vi "Log State.vi"(8 "error in":errorcluster, 10 "Model Status":T3, 11 "Data":T1) -> (0 "error out":errorcluster, 3 "Data out":T1)   [LabVIEW 2015, in "Logger.lvlib"]
uses:
  Logger.lvlib
  Model/TypeDefs/Get Model Status Control.ctl
  TypeDefs/Logger Data.ctl
  TypeDefs/Logger State.ctl
  Model/Model.lvlib
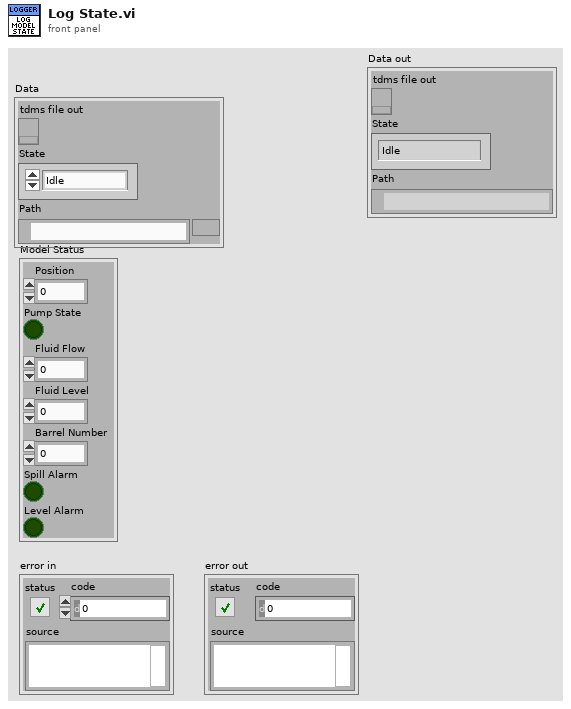
[diagram p1: front panel]
types:
  T1 = typedef "Logger.lvlib/Logger Data.ctl" = cluster{"tdms file out":refnum<k34>, "State":T2, "Path":path}
  T2 = typedef "Logger.lvlib/Logger State.ctl" = enum16{"Idle", "Working"}
  T3 = typedef "Model.lvlib/Get Model Status Control.ctl" = cluster{"Position":dbl, "Pump State":bool, "Fluid Flow":dbl, "Fluid Level":dbl, "Barrel Number":i32, "Spill Alarm":bool, "Level Alarm":bool}
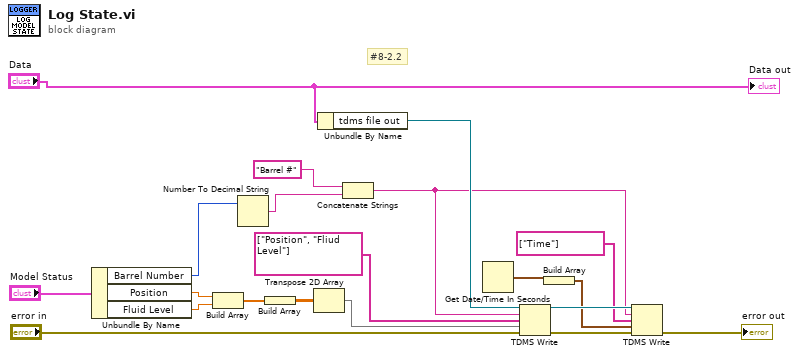
[diagram p0: block diagram]
diagram:
  # "#8-2.2"
  n1 = Unbundle By Name("Model Status") -> ("Barrel Number"=w14:i32, "Position"=w8:dbl, "Fluid Level"=w7:dbl)
  n2 = Build Array(w8, w7) -> (w6:dbl[])
  n3 = Number To Decimal String(number=w14) -> (decimal integer string=w13:string)  [unwired: 1 in]
  n4 = Build Array(w6) -> (w5:dbl[][])
  n5 = Transpose 2D Array(2D array=w5) -> (transposed array=w4:dbl[][])
  n6 = Unbundle By Name("Data") -> ("tdms file out"=w17:refnum<k34>)
  n7 = Concatenate Strings("Barrel #" ("string"), w13) -> (w3:string)
  n8 = Get Date/Time In Seconds() -> (seconds since 1Jan1904=w2:timestamp)
  n9 = TDMS Write(0:w17, 5:w3, 7:string[] ["Position", "Fliud Level"], 9:w4, 11:"error in") -> (4:w11:refnum<k34>, 15:w16:errorcluster)  [unwired: 1 in, 2 out]
  n10 = Build Array(w2) -> (w1:timestamp[])
  n11 = TDMS Write(0:w11, 5:w3, 7:string[] ["Time"], 9:w1, 11:w16) -> (15:→"error out":errorcluster)  [unwired: 1 in, 3 out]
  "Data out" <- "Data"
